vi "Analyze State.vi"(8 "error in (no error)":errorcluster, 11 "Elevator Controller Actor in":refnum<class "Elevator Controller Actor.lvclass">) -> (0 "error out":errorcluster, 3 "Elevator Controller Actor out":refnum<class "Elevator Controller Actor.lvclass">)   [LabVIEW 2019]
uses:
  Elevator Controller Actor.lvclass
  State -Enum.ctl
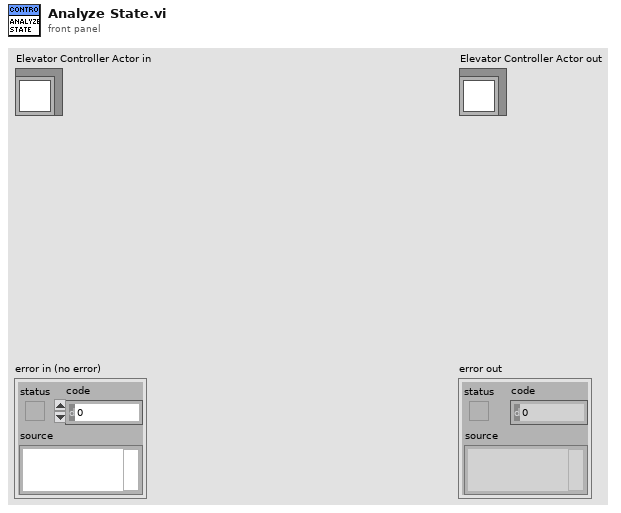
[diagram p1: front panel]
types:
  T1 = typedef "Elevator Controller Actor.lvlib/Elevator Controller Actor.lvclass/State -Enum.ctl" = enum16{"Initial", "Wait for First Request", "Start and Move", "Anaysis", "Continue Travel", "Stop at Floor", "Open and Close Door Sequence", "No Request Remaining", "Emergency Call", "Terminate Process"}
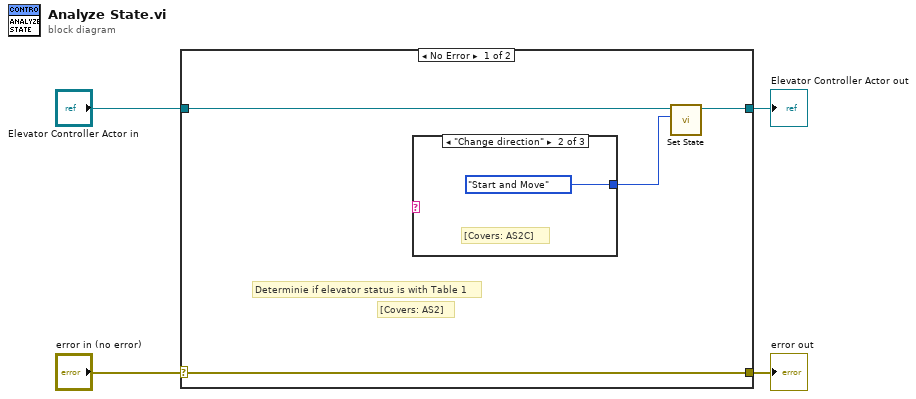
[diagram p0: block diagram]
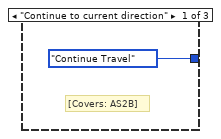
[diagram p2: hidden frame]
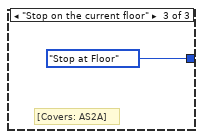
[diagram p3: hidden frame]
diagram:
  n1 = case shown="No Error" "error in (no error)" {
    selector: "error in (no error)" -> [w8 w13]
    tunnel: [w8 w13] -> w3
    tunnel: [w7 w12] -> w1
    tunnel: "Elevator Controller Actor in" -> [w5 w12]
    frame No Error {
      # "[Covers: AS2]"
      # "Determinie if elevator status is with Table 1"
      n2 = case shown="\"Change direction\"" {
        selector: _ -> [_ _ _]
        tunnel: [State_-Enum."Continue Travel" ("States") State_-Enum."Start and Move" ("States") State_-Enum."Stop at Floor" ("States")] -> w6
        frame "Continue to current direction" {
          # "[Covers: AS2B]"
        }
        frame "Change direction" {
          # "[Covers: AS2C]"
        }
        frame "Stop on the current floor" {
          # "[Covers: AS2A]"
        }
      }
      n3 = call "Set State.vi"("States"=w6, "Elevator Controller Actor in"=w5) -> ("Elevator Controller Actor out"=w7:refnum<class "Elevator Controller Actor.lvclass">)  [unwired: 8 in, 1 out]
    }
    frame Error {
    }
  }
  "error out" <- w3
  "Elevator Controller Actor out" <- w1
